vi "setScatterColor.vi"(11 "Features":sgl[][](array[numeric])) -> (3 "3D Plot lvclass Array out":refnum<class "3D Plot Datatype.lvclass">[](array[class]))   [LabVIEW 2023]
uses:
  <vilib>/Math Plots/3D Math Plots/3D Plot/3D Plot Datatype/3D Plot Datatype.lvclass
  <vilib>/Math Plots/3D Math Plots/3D Scatter/3D Scatter Datatype/Public/Plot Helper (Vector).vi
  <vilib>/Math Plots/3D Math Plots/3D Scatter/3D Scatter Datatype/3D Scatter Datatype.lvclass
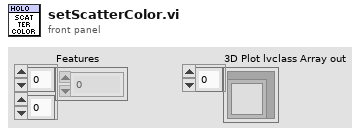
[diagram p1: front panel]
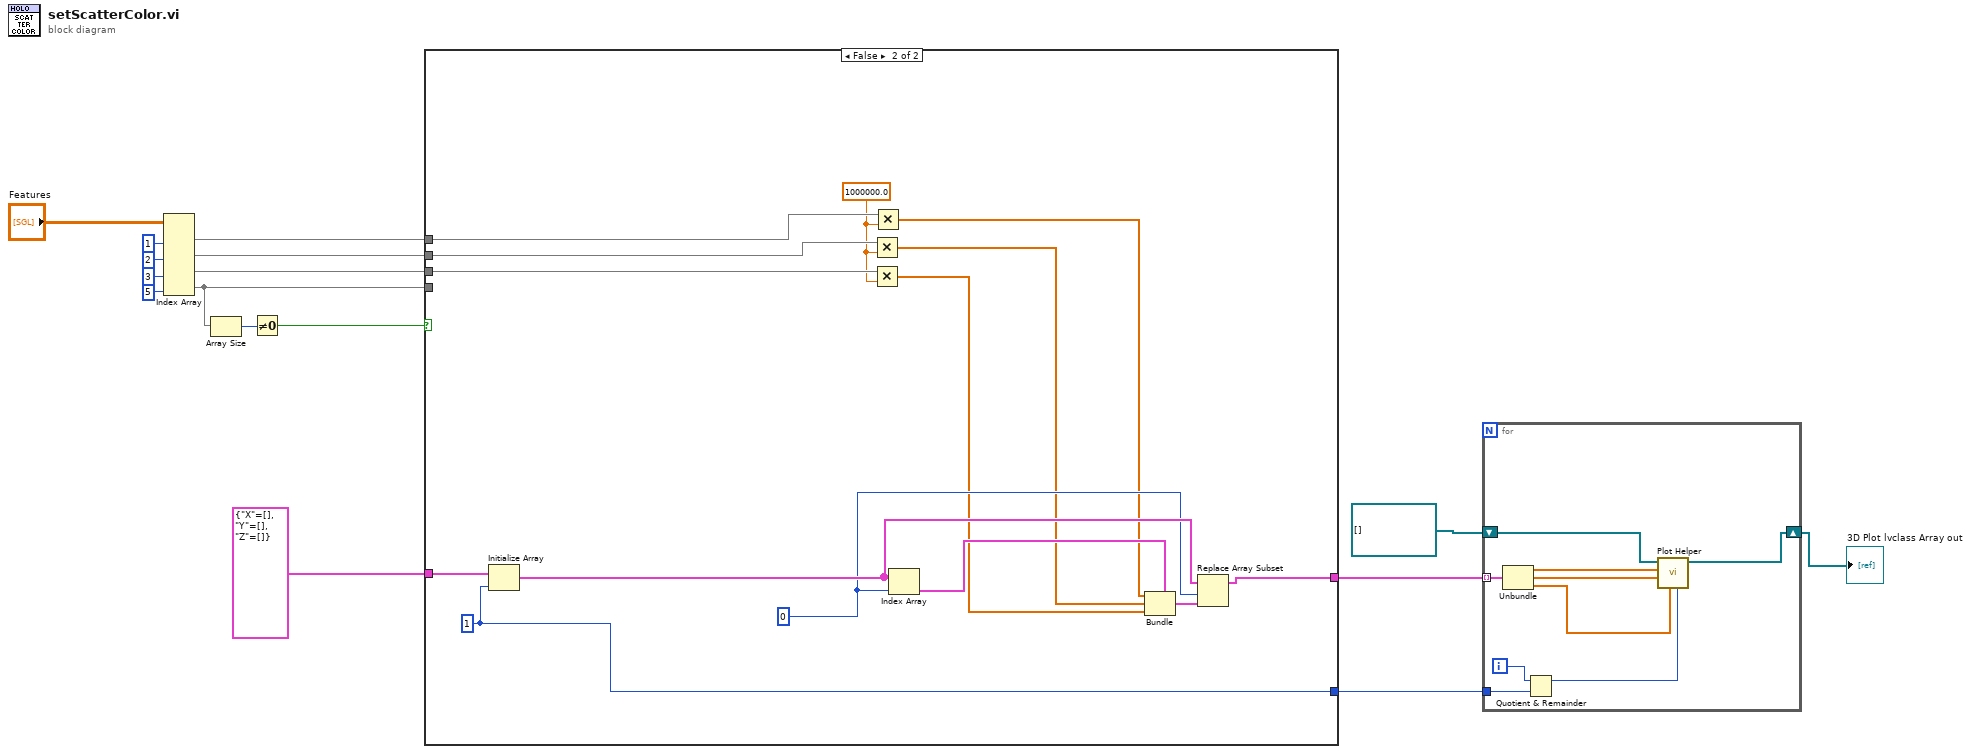
[diagram p0: block diagram]
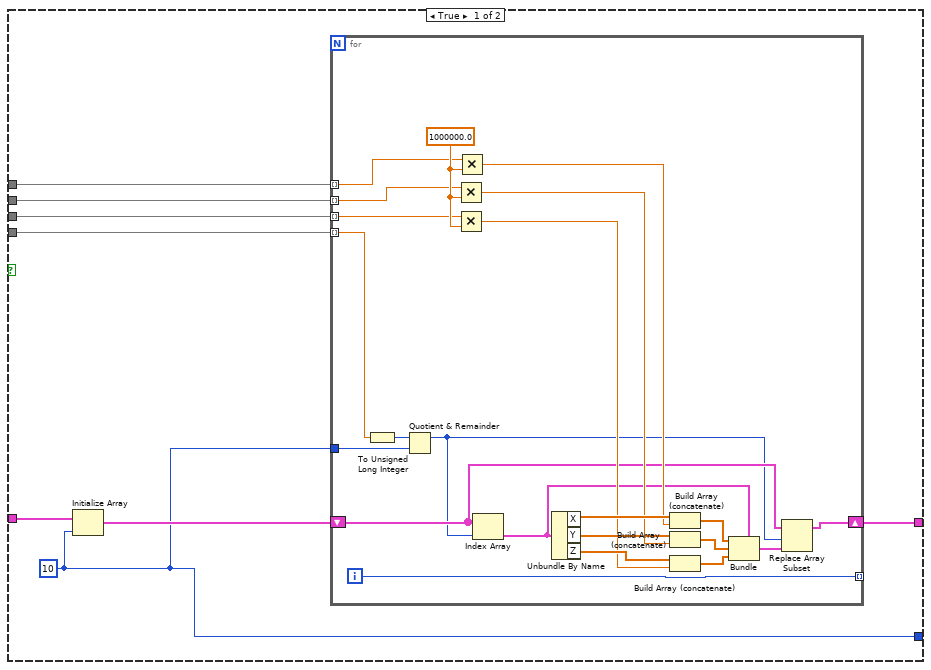
[diagram p2: hidden frame]
diagram:
  n1 = Index Array(array="Features", index (col) #1=1 ("disabled index (col)"), index (col) #2=2 ("index (col)"), index (col) #3=3 ("index (col)"), index (col) #4=5 ("index (col)")) -> (element #1=w11:sgl[], element #2=w10:sgl[], element #3=w13:sgl[], element #4=w7:sgl[])  [unwired: 4 in]
  n2 = Array Size(array=w7) -> (size(s)=w6:i32)
  n3 = Not Equal To 0?(x=w6) -> (x != 0?=w1:bool)
  n4 = case shown="False" w1 {
    tunnel: w13 -> [w24 w60]
    tunnel: w11 -> [w23 w59]
    tunnel: w10 -> [w22 w58]
    tunnel: w7 -> [w21 _]
    tunnel: cluster{"X":sgl[], "Y":sgl[], "Z":sgl[]} {"X"=[], "Y"=[], "Z"=[]} -> [w20 w57]
    tunnel: [w18 w55] -> w4
    tunnel: [w17 w54] -> w2
    frame True {
      w17 = 10 ("dimension size")
      n5 = Initialize Array(w20, w17) -> (w19:cluster{"X":sgl[], "Y":sgl[], "Z":sgl[]}[])
      n6 = for {
        tunnel: w24 -> [w45] mode=indexing
        tunnel: w23 -> [w44] mode=indexing
        tunnel: w22 -> [w43] mode=indexing
        tunnel: w21 -> [w42] mode=indexing
        shift-right: [w26] -> w18
        shift-left: w19 -> [w29]
        tunnel: w17 -> [w40]
        tunnel: [w25] -> _ mode=indexing
        i -> [w25]
        w46 = 1000000.0
        n7 = To Unsigned Long Integer(number=w42) -> (unsigned 32bit integer=w41:u32)
        n8 = Quotient & Remainder(x=w41, y=w40) -> (x-y*floor(x/y)=w27:u32)  [unwired: 1 out]
        n9 = Multiply(x=w43, y=w46) -> (x*y=w37:dbl)
        n10 = Multiply(x=w45, y=w46) -> (x*y=w34:dbl)
        n11 = Multiply(x=w44, y=w46) -> (x*y=w38:dbl)
        n12 = Index Array(array=w29, index=w27) -> (element=w33:cluster{"X":sgl[], "Y":sgl[], "Z":sgl[]})
        n13 = Unbundle By Name(w33) -> ("X"=w39:sgl[], "Y"=w36:sgl[], "Z"=w35:sgl[])
        n14 = Build Array (concatenate)(w39, w38) -> (w32:dbl[])
        n15 = Build Array (concatenate)(w36, w37) -> (w31:dbl[])
        n16 = Build Array (concatenate)(w35, w34) -> (w30:dbl[])
        n17 = Bundle(cluster=w33, "X"=w32, "Y"=w31, "Z"=w30) -> (w28:cluster{"X":sgl[], "Y":sgl[], "Z":sgl[]})
        n18 = Replace Array Subset(array=w29, new element=w28, index=w27) -> (w26:cluster{"X":sgl[], "Y":sgl[], "Z":sgl[]}[])
      }
    }
    frame False {
      w50 = 0 ("index")
      w53 = 1000000.0
      w54 = 1 ("dimension size")
      n19 = Initialize Array(w57, w54) -> (w56:cluster{"X":sgl[], "Y":sgl[], "Z":sgl[]}[])
      n20 = Multiply(x=w58, y=w53) -> (x*y=w48:dbl[])
      n21 = Multiply(x=w60, y=w53) -> (x*y=w47:dbl[])
      n22 = Multiply(x=w59, y=w53) -> (x*y=w49:dbl[])
      n23 = Index Array(array=w56, index=w50) -> (element=w52:cluster{"X":sgl[], "Y":sgl[], "Z":sgl[]})
      n24 = Bundle(cluster=w52, "X"=w49, "Y"=w48, "Z"=w47) -> (w51:cluster{"X":sgl[], "Y":sgl[], "Z":sgl[]})
      n25 = Replace Array Subset(array=w56, new element=w51, index=w50) -> (w55:cluster{"X":sgl[], "Y":sgl[], "Z":sgl[]}[])
    }
  }
  n26 = for {
    tunnel: w4 -> [w69] mode=indexing
    shift-right: [w65] -> w8
    shift-left: refnum<class "3D Plot Datatype.lvclass">[] [] ("3D Plot lvclass Array out") -> [w64]
    tunnel: w2 -> [w62]
    i -> [w63]
    n27 = Unbundle(w69) -> ("X"=w68:sgl[], "Y"=w67:sgl[], "Z"=w66:sgl[])
    n28 = Quotient & Remainder(x=w63, y=w62) -> (x-y*floor(x/y)=w61:i32)  [unwired: 1 out]
    n29 = call-poly <vilib>:"Plot Helper.vi"("Plot ID"=w61, "z vector"=w66, "y vector"=w67, "x vector"=w68, "3D Plot lvclass Array in"=w64) -> ("3D Plot lvclass Array out"=w65:refnum<class "3D Plot Datatype.lvclass">[])  [unwired: 1 in, 5 out]
  }
  "3D Plot lvclass Array out" <- w8
